vi "Start_Stop Aq.vi"(8 "error in (no error)":errorcluster, 10 "Start/Stop AQ":bool, 11 "Businness Logic in":refnum<class "Businness Logic.lvclass">) -> (0 "error out":errorcluster, 3 "Businness Logic out":refnum<class "Businness Logic.lvclass">)   [LabVIEW 2020, in "Businness Logic.lvlib" / "Businness Logic.lvclass"]
uses:
  Businness Logic.lvclass
  Businness Logic.lvclass/Businness Logic.ctl
  Acquisition/Acquisition Messages/Start_Stop AQ Msg/Start_Stop AQ Msg.lvclass
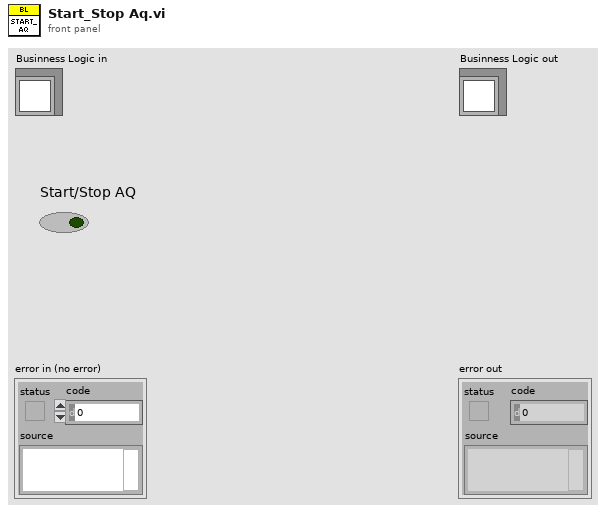
[diagram p1: front panel]
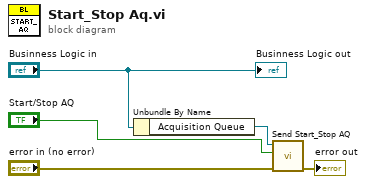
[diagram p0: block diagram]
diagram:
  n1 = Unbundle By Name("Businness Logic in") -> ("Acquisition Queue"=w3:refnum<class "Message Enqueuer.lvclass">)
  n2 = call "Send Start_Stop AQ.vi"("error in (no error)"="error in (no error)", "Start_Stop"="Start/Stop AQ", "Message Enqueuer"=w3) -> ("error out"=→"error out":errorcluster)  [unwired: 7 in, 1 out]
  "Businness Logic out" <- "Businness Logic in"
